vi "CMC_Boolean_String_Controls_Indicators.vi"() -> ()   [LabVIEW 2013]
panel:
  out "Indicator":string
  in  "Control":string
  out "Indicator":bool
  in  "Control":bool
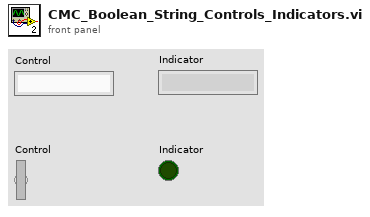
[diagram p1: front panel]
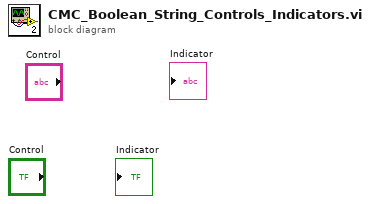
[diagram p0: block diagram]
diagram:
